vi "Compare.vi"(8 "error in (no error)":errorcluster, 10 "Hand in 2":refnum<class "Hand.lvclass">, 11 "Hand in":refnum<class "Hand.lvclass">) -> (0 "error out":errorcluster, 2 "Higher?":bool, 3 "Hand out":refnum<class "Hand.lvclass">)   [LabVIEW 2020, in "Hand.lvclass"]
uses:
  Hand.lvclass
  Hand.lvclass/Hand.ctl
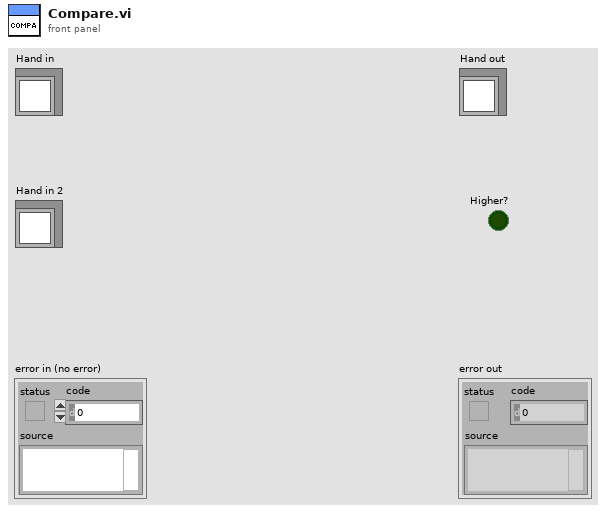
[diagram p1: front panel]
types:
  T1 = enum16{"High Card", "One Pair", "Two Pairs", "Three of a Kind", "Full House", "Four of a Kind", "Five of a Kind"}
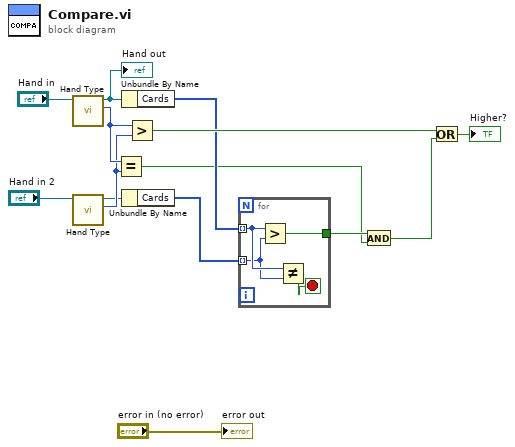
[diagram p0: block diagram]
diagram:
  n1 = call "Hand Type.vi"("Hand In"="Hand in") -> ("Score"=w10:T1, "Hand Out"=w8:refnum<class "Hand.lvclass">)  [unwired: 8 in, 1 out]
  "Hand out" <- w8
  n2 = call "Hand Type.vi"("Hand In"="Hand in 2") -> ("Score"=w9:T1, "Hand Out"=w6:refnum<class "Hand.lvclass">)  [unwired: 8 in, 1 out]
  n3 = Equal?(x=w10, y=w9) -> (x = y?=w1:bool)
  n4 = Unbundle By Name(w8) -> ("Cards"=w7:u8[])
  n5 = Unbundle By Name(w6) -> ("Cards"=w5:u8[])
  n6 = Greater?(x=w10, y=w9) -> (0:w11:bool)
  n7 = for {
    tunnel: w7 -> [w17] mode=indexing
    tunnel: w5 -> [w16] mode=indexing
    tunnel: [w18] -> w3
    stop <- w15 stop-if-true
    n8 = Greater?(x=w17, y=w16) -> (0:w18:bool)
    n9 = Not Equal?(x=w17, y=w16) -> (x != y?=w15:bool)
  }
  n10 = And(x=w3, y=w1) -> (x .and. y?=w2:bool)
  n11 = Or(x=w11, y=w2) -> (x .or. y?=→"Higher?":bool)
  "error out" <- "error in (no error)"
